vi "Client 1.vi"(8 "error in (no error)":errorcluster, 10 "Queue Name":string) -> (0 "error out":errorcluster)   [LabVIEW 2011]
doc: "One instance of the Client in the QDMH Client - Server example. This demonstration illustrates one way to take the existing QDMH and extend funtionality. Multiple clients can \"connect\" to the server. Examine the block diagram to see how the server keeps track of which client has made a connection. This is an illustration of leveraging the flexiblitiy of named queues.\n\nAAL 9/09"
uses:
  Shared/QDMH Poly VIs/QDMH POLY Enqueue String.vi
  Shared/QDMH Poly VIs/QDMH POLY Enqueue Cluster.vi
panel:
  in  "Get Data":bool
  out "Message Display":string
  in  "Cancel":bool
  in  "OK":bool
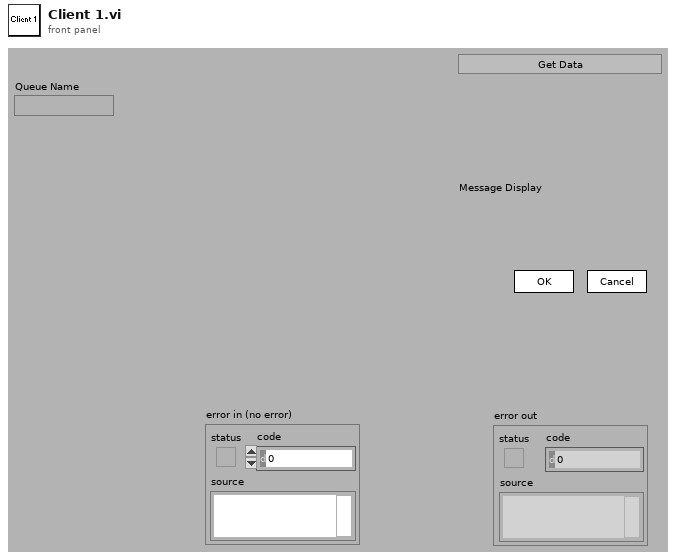
[diagram p1: front panel]
types:
  T1 = cluster{"Operator Name":string, "Current VI's Path":path, "Current VI's  Directory":path, "Queue Names":string[], "# VIs Launched":i32}
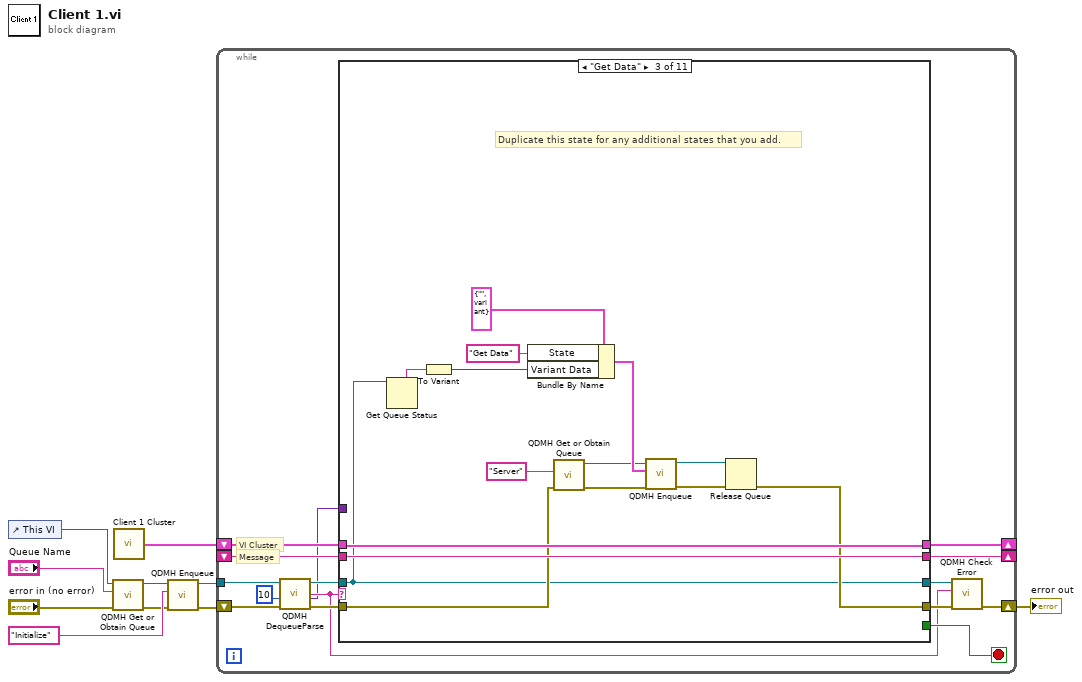
[diagram p0: block diagram]
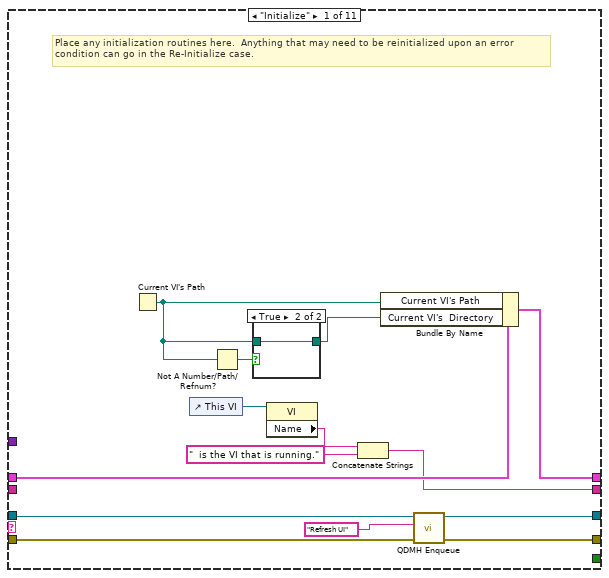
[diagram p2: hidden frame]
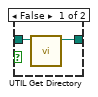
[diagram p3: hidden frame]
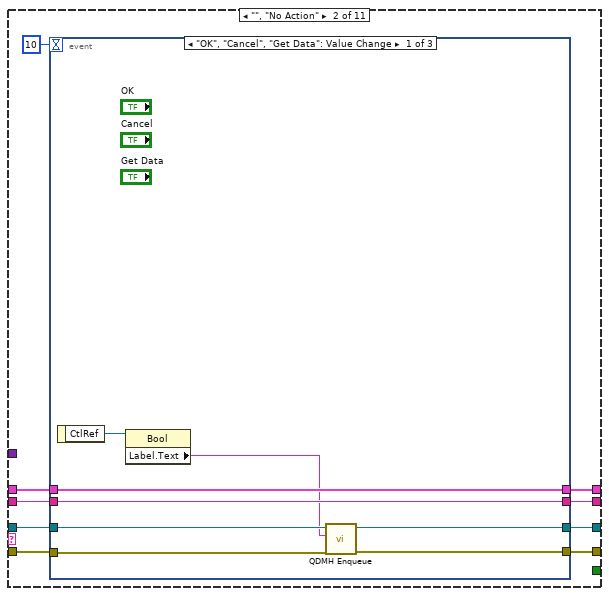
[diagram p4: hidden frame]
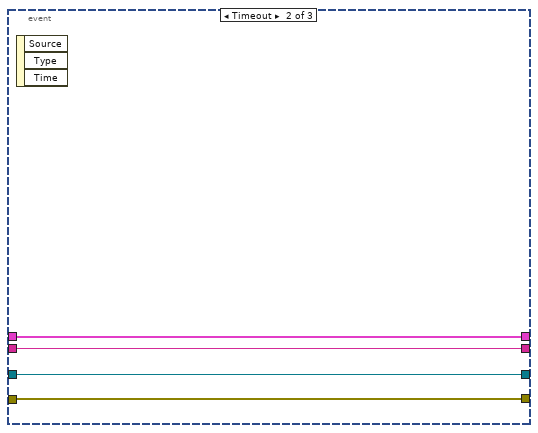
[diagram p5: hidden frame]
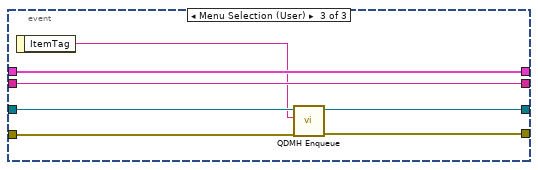
[diagram p6: hidden frame]
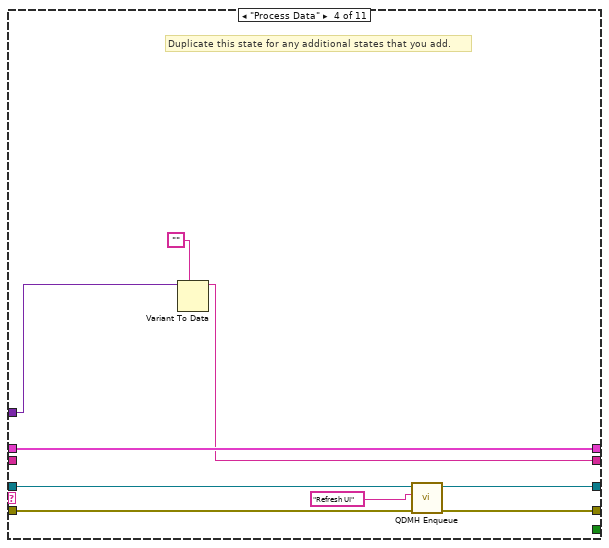
[diagram p7: hidden frame]
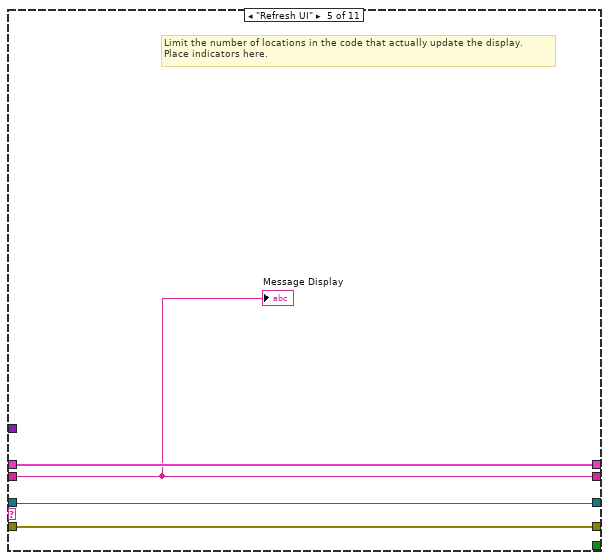
[diagram p8: hidden frame]
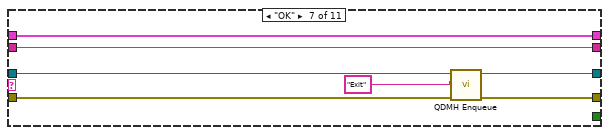
[diagram p10: hidden frame]
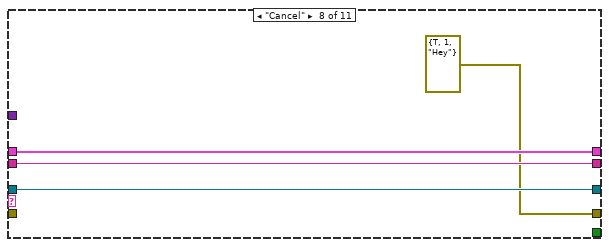
[diagram p11: hidden frame]
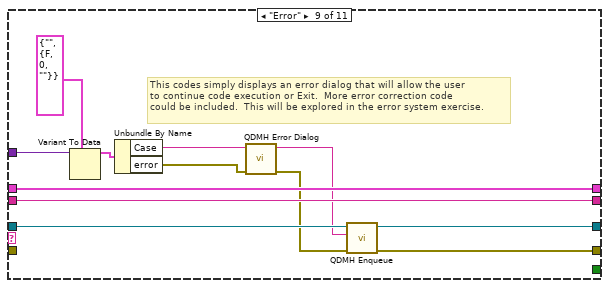
[diagram p12: hidden frame]
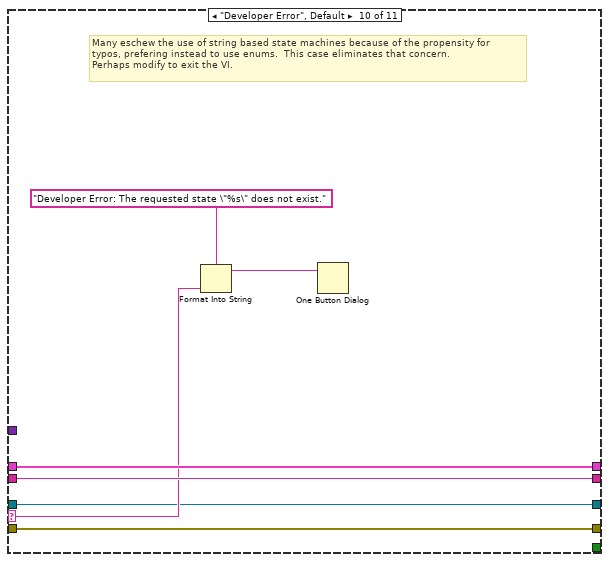
[diagram p13: hidden frame]
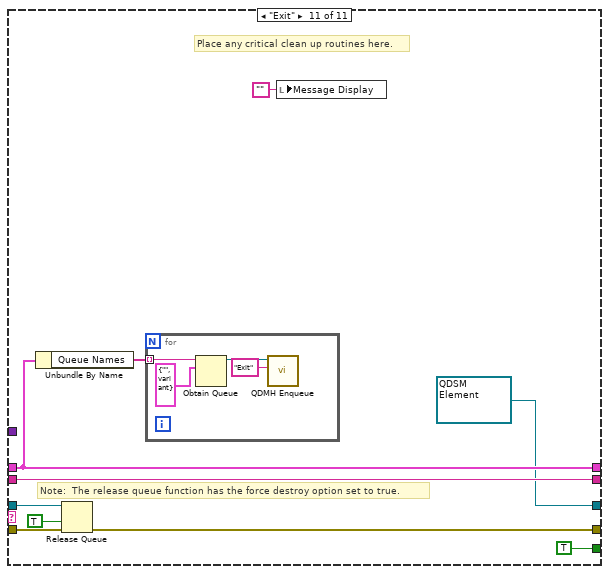
[diagram p14: hidden frame]
diagram:
  n1 = control-ref of="This VI"() -> (w1:refnum<vi>)
  n2 = call "QDMH Get or Obtain Queue.vi"("error in (no error)"="error in (no error)", "Queue Name"="Queue Name", "VI Refnum"=w1) -> ("error out"=w4:errorcluster, "queue out"=w5:refnum<queue>)  [unwired: 7 out]
  n3 = call "Client 1 Cluster.vi"() -> ("Cluster"=w10:T1)
  n4 = call-poly "QDMH Enqueue.vi"("error in (no error)"=w4, "State"="Initialize" ("element"), "queue"=w5) -> ("error out"=w2:errorcluster, "queue out"=w3:refnum<queue>)  [unwired: 7 out]
  n5 = while {
    tunnel: w3 -> [w20]
    shift-left: w10 -> [w21]
    shift-right: [w22] -> _
    shift-left: _ -> [w23]
    shift-right: [w24] -> _
    shift-right: [w14] -> w8
    shift-left: w2 -> [w16]
    stop <- w25 stop-if-true
    # "VI Cluster"
    # "Message"
    n6 = call "QDMH DequeueParse.vi"("error in (no error)"=w16, "Timeout"=10 ("ms timeout (-1)"), "queue"=w20) -> ("error out"=w17:errorcluster, "Variant Data"=w11:variant, "State"=w12:string, "queue out"=w18:refnum<queue>)  [unwired: 5 out]
    n7 = case shown="\"Get Data\"" w12 {
      selector: w12 -> [_ _ _ _ _ _ _ _ _ w129 _]
      tunnel: w18 -> [w35 w51 w71 w90 w96 w99 w109 w111 w123 w126 w139]
      tunnel: [_ _ _ _ _ _ _ _ _ _ TRUE] -> w25
      tunnel: [w33 w44 w76 w91 w97 w102 w108 w113 w125 w132 w141] -> w24
      tunnel: w23 -> [_ w45 w76 _ w97 w102 w108 w113 w125 w132 w141]
      tunnel: [w38 w46 w85 w94 w98 w101 w107 w112 w124 w131 w136] -> w22
      tunnel: w21 -> [w39 w47 w85 w94 w98 w101 w107 w112 w124 w131 w136]
      tunnel: w17 -> [w37 w50 w75 w88 w95 w100 w106 _ _ w128 w138]
      tunnel: [w36 w49 w72 w87 w95 w100 w105 errorcluster {"status"=TRUE, "code"=1, "source"="Hey"} ("error out") w122 w128 w133] -> w15
      tunnel: [w28 w43 w71 w89 w96 w99 w103 w111 w121 w126 refnum<queue> refnum ("queue out")] -> w13
      tunnel: w11 -> [_ _ _ w93 _ _ _ _ w119 _ _]
      frame "Initialize" {
        # "Place any initialization routines here.  Anything that may need to be reinitialized upon an error\ncondition can go in the Re-Initialize case."
        n8 = Current VI's Path() -> (path=w26:path)
        n9 = control-ref of="This VI"() -> (w32:refnum<vi>)
        n10 = Not A Number/Path/Refnum?(number/path/refnum=w26) -> (NaN/Path/Refnum?=w27:bool)
        n11 = case shown="True" w27 {
          tunnel: w26 -> [w41 w42]
          tunnel: [w40 w42] -> w30
          frame False {
            n12 = call "UTIL Get Directory.vi"("Path In"=w41) -> ("Directory Out"=w40:path)  [unwired: 1 in, 9 out]
          }
          frame True {
          }
        }
        n13 = property class="VI"(reference=w32) -> ("Name"=w31:string)  [unwired: 1 in, 2 out]
        n14 = Concatenate Strings(w31, "  is the VI that is running." ("string")) -> (w33:string)
        n15 = Bundle By Name(cluster=w39, "Current VI's Path"=w26, "Current VI's  Directory"=w30) -> (w38:T1)
        n16 = call-poly "QDMH Enqueue.vi"("error in (no error)"=w37, "State"="Refresh UI" ("New State"), "queue"=w35) -> ("error out"=w36:errorcluster, "queue out"=w28:refnum<queue>)  [unwired: 7 out]
      }
      frame "", "No Action" {
        n17 = event shown="[0] \"OK\", \"Cancel\", \"Get Data\": Value Change" {
          selector: _ -> [_ _ _]
          dyn-events: _ -> [_ _ _]
          timeout: 10 -> [_ _ _]
          tunnel: w51 -> [w58 w60 w70]
          tunnel: [w57 w63 w68] -> w49
          tunnel: w50 -> [w56 w63 w69]
          tunnel: w47 -> [w55 w62 w67]
          tunnel: [w55 w62 w67] -> w46
          tunnel: w45 -> [w54 w61 w66]
          tunnel: [w54 w61 w66] -> w44
          tunnel: [w52 w60 w64] -> w43
          event "OK", "Cancel", "Get Data": Value Change {
            n18 = event-data() -> ("CtlRef"=w59:refnum<vi>)  [unwired: 1 out]
            n19 = property class="Bool"(reference=w59) -> ("Label.Text"=w53:string)  [unwired: 1 in, 2 out]
            n20 = call-poly "QDMH Enqueue.vi"("error in (no error)"=w56, "State"=w53, "queue"=w58) -> ("error out"=w57:errorcluster, "queue out"=w52:refnum<queue>)  [unwired: 7 out]
          }
          event Timeout {
            n21 = event-data() -> ()  [unwired: 4 out]
          }
          event Menu Selection (User) {
            n22 = event-data() -> ("ItemTag"=w65:string)  [unwired: 1 out]
            n23 = call-poly "QDMH Enqueue.vi"("error in (no error)"=w69, "State"=w65, "queue"=w70) -> ("error out"=w68:errorcluster, "queue out"=w64:refnum<queue>)  [unwired: 7 out]
          }
        }
      }
      frame "Get Data" {
        # "Duplicate this state for any additional states that you add."
        n24 = Get Queue Status(queue=w71) -> (queue name=w83:string)  [unwired: 1 in, 8 out]
        n25 = To Variant(anything=w83) -> (Variant=w84:variant)
        n26 = Bundle By Name(cluster=cluster{"State":string, "Variant Data":variant} {"State"="", "Variant Data"=variant} ("QDSM Element"), "State"="Get Data" ("element"), "Variant Data"=w84) -> (w79:cluster{"State":string, "Variant Data":variant})
        n27 = call "QDMH Get or Obtain Queue.vi"("error in (no error)"=w75, "Queue Name"="Server" ("name (unnamed)")) -> ("error out"=w77:errorcluster, "queue out"=w78:refnum<queue>)  [unwired: 1 in, 7 out]
        n28 = call-poly "QDMH Enqueue.vi"("error in (no error)"=w77, "QDSM Element"=w79, "queue"=w78) -> ("error out"=w80:errorcluster, "queue out"=w81:refnum<queue>)  [unwired: 7 out]
        n29 = Release Queue(queue=w81, error in (no error)=w80) -> (error out=w72:errorcluster)  [unwired: 3 out]
      }
      frame "Process Data" {
        # "Duplicate this state for any additional states that you add."
        n30 = Variant To Data(type="", Variant=w93) -> (data=w91:string)  [unwired: 1 in, 1 out]
        n31 = call-poly "QDMH Enqueue.vi"("error in (no error)"=w88, "State"="Refresh UI", "queue"=w90) -> ("error out"=w87:errorcluster, "queue out"=w89:refnum<queue>)  [unwired: 7 out]
      }
      frame "Refresh UI" {
        # "Limit the number of locations in the code that actually update the display.\nPlace indicators here."
        "Message Display" <- w97
      }
      frame "<duplicate me for new states >" {
        # "Duplicate this state for any additional states that you add."
      }
      frame "OK" {
        n32 = call-poly "QDMH Enqueue.vi"("error in (no error)"=w106, "State"="Exit" ("New State"), "queue"=w109) -> ("error out"=w105:errorcluster, "queue out"=w103:refnum<queue>)  [unwired: 7 out]
      }
      frame "Cancel" {
      }
      frame "Error" {
        # "This codes simply displays an error dialog that will allow the user\nto continue code execution or Exit.  More error correction code\ncould be included.  This will be explored in the error system exercise."
        n33 = Variant To Data(type=cluster{"Case":string, "error":errorcluster} {"Case"="", "error"={"status"=FALSE, "code"=0, "source"=""}} ("QDSM Element"), Variant=w119) -> (data=w118:cluster{"Case":string, "error":errorcluster})  [unwired: 1 in, 1 out]
        n34 = Unbundle By Name(w118) -> ("Case"=w117:string, "error"=w116:errorcluster)
        n35 = call "QDMH Error Dialog.vi"("error"=w116, "Case Error Occured"=w117) -> ("error out (no error)"=w114:errorcluster, "Case to Execute"=w115:string)  [unwired: 8 out]
        n36 = call-poly "QDMH Enqueue.vi"("error in (no error)"=w114, "State"=w115, "queue"=w123) -> ("error out"=w122:errorcluster, "queue out"=w121:refnum<queue>)  [unwired: 7 out]
      }
      frame "Developer Error", Default {
        # "Many eschew the use of string based state machines because of the propensity for\ntypos, prefering instead to use enums.  This case eliminates that concern.\nPerhaps modify to exit the VI."
        n37 = Format Into String(format string="Developer Error: The requested state \"%s\" does not exist." ("message"), w129) -> (resulting string=w127:string)  [unwired: 2 in, 1 out]
        n38 = One Button Dialog(message=w127) -> ()  [unwired: 2 out]
      }
      frame "Exit" {
        # "Note:  The release queue function has the force destroy option set to true."
        # "Place any critical clean up routines here."
        n39 = Unbundle By Name(w136) -> ("Queue Names"=w134:string[])
        n40 = Release Queue(queue=w139, force destroy? (F)=TRUE, error in (no error)=w138) -> (error out=w133:errorcluster)  [unwired: 2 out]
        n41 = for {
          tunnel: w134 -> [w146] mode=indexing
          n42 = Obtain Queue(name (unnamed)=w146, element data type=cluster{"State":string, "Variant Data":variant} {"State"="", "Variant Data"=variant} ("QDSM Element")) -> (queue out=w145:refnum<queue>)  [unwired: 3 in, 2 out]
          n43 = call-poly "QDMH Enqueue.vi"("State"="Exit" ("element"), "queue"=w145) -> ()  [unwired: 1 in, 9 out]
        }
        n44 = local write "Message Display"("") -> ()
      }
    }
    n45 = call "QDMH Check Error.vi"("error in (no error)"=w15, "Case"=w12, "queue"=w13) -> ("error out"=w14:errorcluster)  [unwired: 1 in, 7 out]
  }
  "error out" <- w8
